vi "set trigger.vi"(8 "error in (no error)":errorcluster, 9 "channel2":u16, 10 "channel1":u16, 11 "sampleperiod":u16) -> (0 "error out":errorcluster)   [LabVIEW 2015, in "SCANalone4x64.lvlib"]
doc: "__declspec(dllimport) void __stdcall set_trigger(unsigned short sampleperiod, unsigned short channel1, unsigned short channel2);"
uses:
  <userlib>/SCANalone4x64/SCANalone4x64.lvlib
  <userlib>/SCANalone4x64/SCANalone4x64.dll
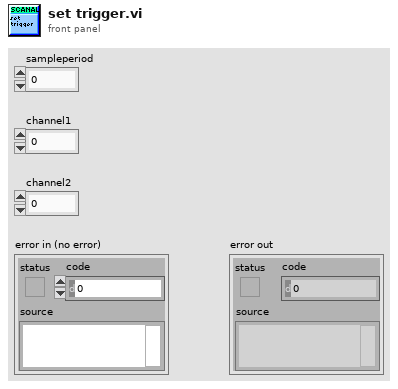
[diagram p1: front panel]
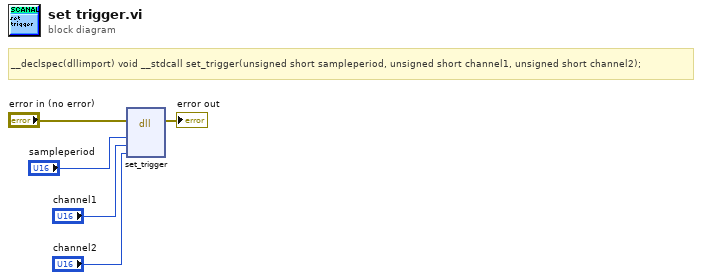
[diagram p0: block diagram]
diagram:
  # "__declspec(dllimport) void __stdcall set_trigger(unsigned short sampleperiod, unsigned short channel1, unsigned short channel2);"
  n1 = dll-call lib="C:/Program Files/National Instruments/LabVIEW 2015/user.lib/SCANalone4x64/SCANalone4x64.*" fn="set_trigger"(error in="error in (no error)", "sampleperiod"="sampleperiod", "channel1"="channel1", "channel2"="channel2") -> (error out=→"error out":errorcluster)  [unwired: 6 in, 1 out]
